vi "SMSsendCommand.vi"(0 "HULK SMS address in":refnum<visa-resource-name>, 1 "SMS controls":T1, 5 "error in":errorcluster, 6 "MID field value":dbl, 7 "Voltage limit":dbl, 8 "MAX field value":dbl, 9 "Set heater (V)":dbl, 10 "RAMP rate":dbl, 11 "Field constant (Tesla/Amp)":dbl) -> (14 "HULK SMS address out":refnum<visa-resource-name>, 17 "return count":u32, 19 "error out":errorcluster)   [LabVIEW 2017]
uses:
  SMScontrols.ctl
panel:
  out "concatenated string":string
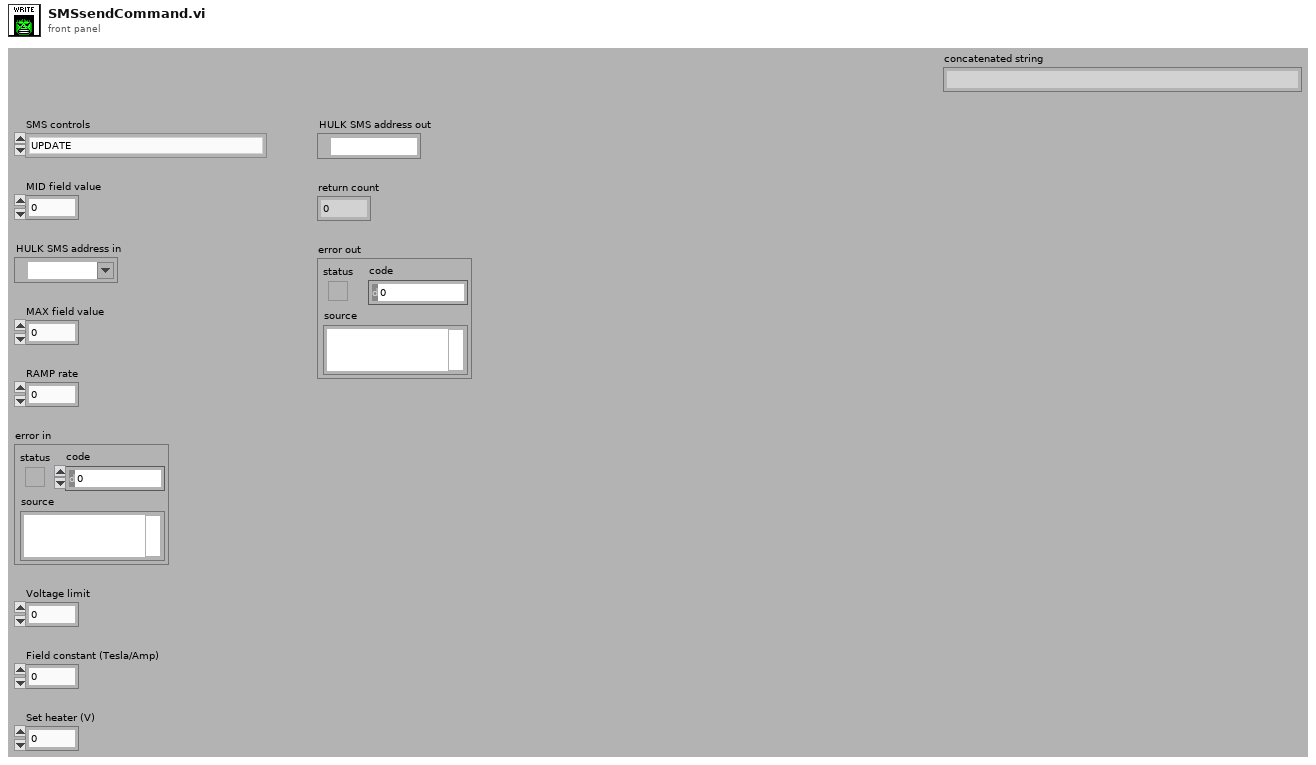
[diagram p1: front panel]
types:
  T1 = typedef "SMScontrols.ctl" = enum16{"UPDATE", "GET OUTPUT", "RAMP ZERO", "RAMP MID", "RAMP MAX", "RAMP STATUS", "PAUSE OFF", "PAUSE ON", "HEATER OFF", "HEATER ON", "TESLA OFF", "TESLA ON", "DIRECTION +", "DIRECTION -", "DIRECTION 0", "SET MID", "SET MAX", "SET RAMP", "SET LIMIT", "SET TPA", "SET HEATER"}
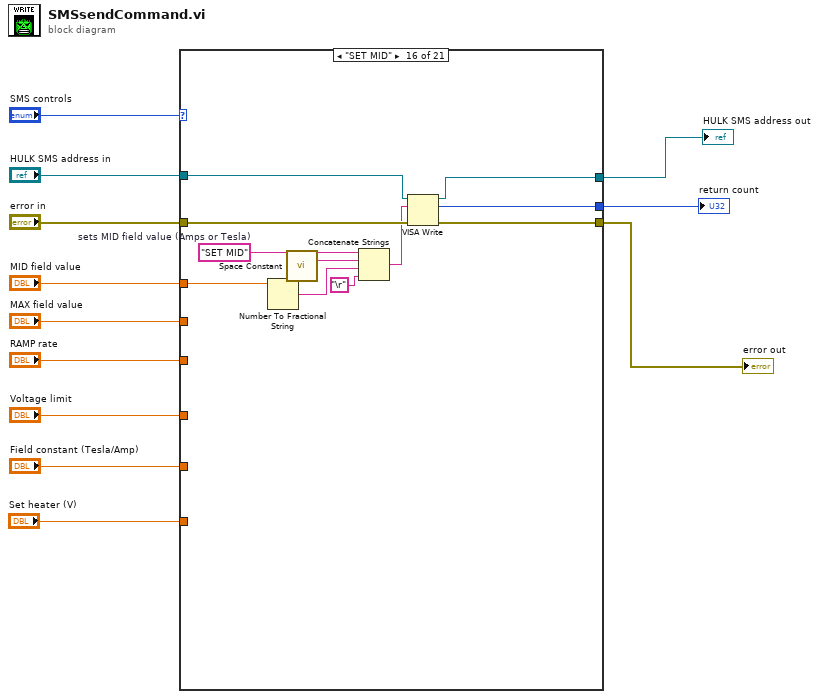
[diagram p0: block diagram]
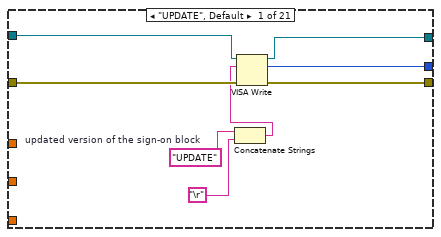
[diagram p2: hidden frame]
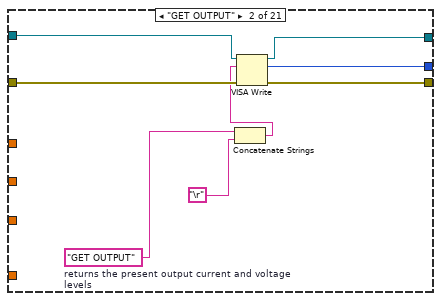
[diagram p3: hidden frame]
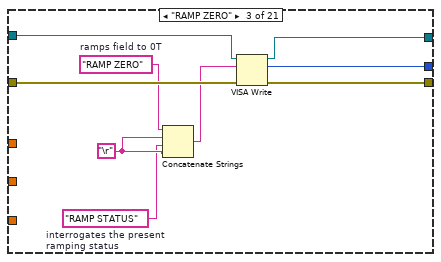
[diagram p4: hidden frame]
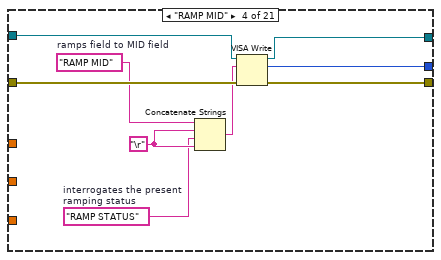
[diagram p5: hidden frame]
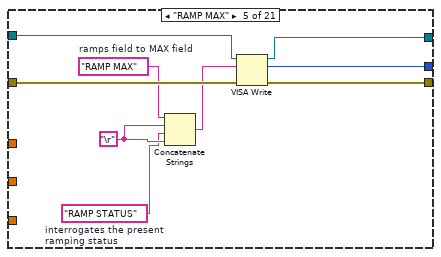
[diagram p6: hidden frame]
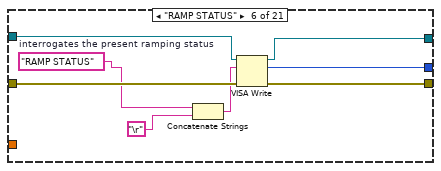
[diagram p7: hidden frame]
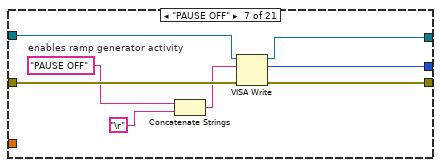
[diagram p8: hidden frame]
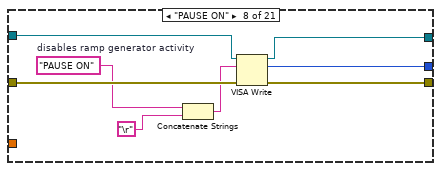
[diagram p9: hidden frame]
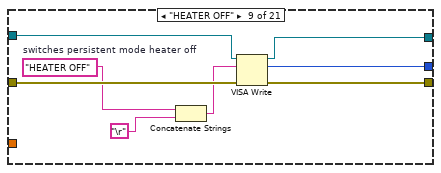
[diagram p10: hidden frame]
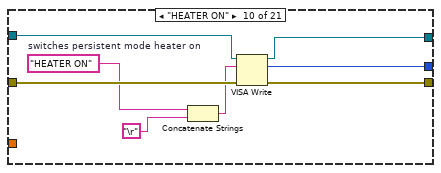
[diagram p11: hidden frame]
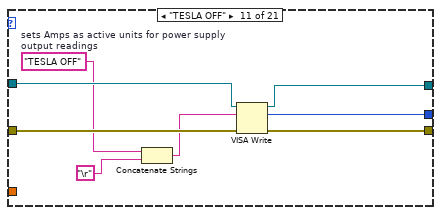
[diagram p12: hidden frame]
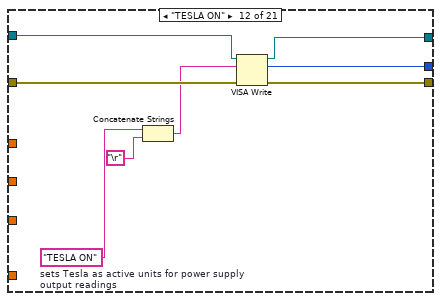
[diagram p13: hidden frame]
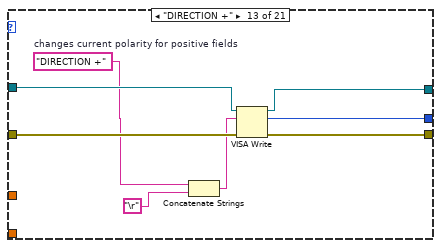
[diagram p14: hidden frame]
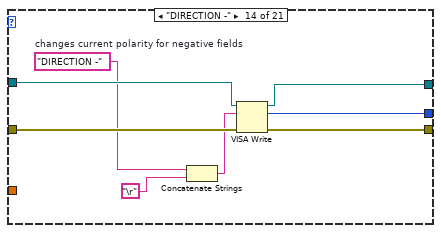
[diagram p15: hidden frame]
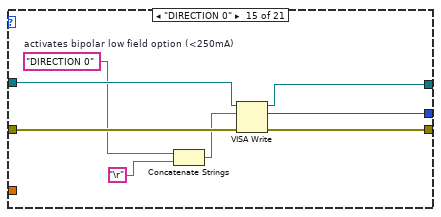
[diagram p16: hidden frame]
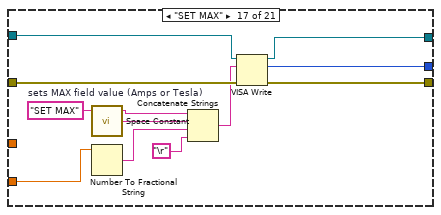
[diagram p17: hidden frame]
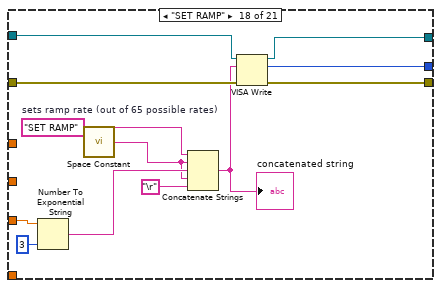
[diagram p18: hidden frame]
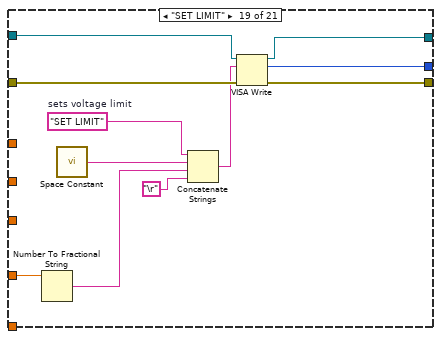
[diagram p19: hidden frame]
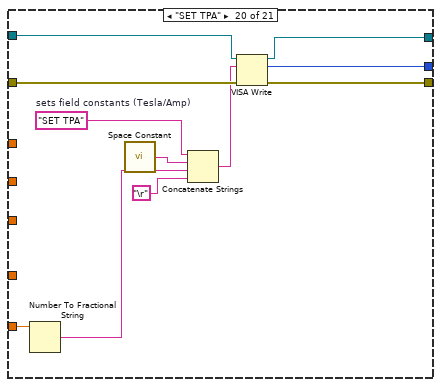
[diagram p20: hidden frame]
diagram:
  n1 = case shown="\"SET MID\"" "SMS controls" {
    tunnel: "HULK SMS address in" -> [w20 w28 w37 w46 w55 w63 w71 w79 w87 w95 w103 w111 w119 w127 w135 w146 w157 w169 w180 w191 w202]
    tunnel: [w19 w27 w36 w45 w54 w62 w70 w78 w86 w94 w102 w110 w118 w126 w134 w145 w156 w168 w179 w190 w201] -> w3
    tunnel: "error in" -> [w18 w26 w35 w44 w53 w61 w69 w77 w85 w93 w101 w109 w117 w125 w133 w144 w155 w167 w178 w189 w200]
    tunnel: [w17 w25 w34 w43 w52 w60 w68 w76 w84 w92 w100 w108 w116 w124 w132 w143 w154 w166 w177 w188 w199] -> w5
    tunnel: [w16 w24 w33 w42 w51 w59 w67 w75 w83 w91 w99 w107 w115 w123 w131 w142 w153 w165 w176 w187 w198] -> w6
    tunnel: "MID field value" -> [_ _ _ _ _ _ _ _ _ _ _ _ _ _ _ w138 _ _ _ _ _]
    tunnel: "MAX field value" -> [_ _ _ _ _ _ _ _ _ _ _ _ _ _ _ _ w148 _ _ _ _]
    tunnel: "RAMP rate" -> [_ _ _ _ _ _ _ _ _ _ _ _ _ _ _ _ _ w161 _ _ _]
    tunnel: "Voltage limit" -> [_ _ _ _ _ _ _ _ _ _ _ _ _ _ _ _ _ _ w171 _ _]
    tunnel: "Field constant (Tesla/Amp)" -> [_ _ _ _ _ _ _ _ _ _ _ _ _ _ _ _ _ _ _ w182 _]
    tunnel: "Set heater (V)" -> [_ _ _ _ _ _ _ _ _ _ _ _ _ _ _ _ _ _ _ _ w193]
    frame "UPDATE", Default {
      w15 = "UPDATE"  # updated version of the sign-on block
      n2 = Concatenate Strings(w15, "\r") -> (w13:string)
      n3 = VISA Write(VISA resource name=w20, write buffer=w13, error in (no error)=w18) -> (VISA resource name out=w17:refnum<visa-resource-name>, return count=w16:u32, error out=w19:errorcluster)
    }
    frame "GET OUTPUT" {
      w21 = "GET OUTPUT"  # returns the present output current and voltage levels
      n4 = Concatenate Strings(w21, "\r") -> (w22:string)
      n5 = VISA Write(VISA resource name=w28, write buffer=w22, error in (no error)=w26) -> (VISA resource name out=w25:refnum<visa-resource-name>, return count=w24:u32, error out=w27:errorcluster)
    }
    frame "RAMP ZERO" {
      w29 = "RAMP STATUS"  # interrogates the present ramping status
      w30 = "\r"
      w32 = "RAMP ZERO"  # ramps field to 0T
      n6 = Concatenate Strings(w32, w30, w29, w30) -> (w31:string)
      n7 = VISA Write(VISA resource name=w37, write buffer=w31, error in (no error)=w35) -> (VISA resource name out=w34:refnum<visa-resource-name>, return count=w33:u32, error out=w36:errorcluster)
    }
    frame "RAMP MID" {
      w38 = "RAMP STATUS"  # interrogates the present ramping status
      w39 = "\r"
      w41 = "RAMP MID"  # ramps field to MID field
      n8 = Concatenate Strings(w41, w39, w38, w39) -> (w40:string)
      n9 = VISA Write(VISA resource name=w46, write buffer=w40, error in (no error)=w44) -> (VISA resource name out=w43:refnum<visa-resource-name>, return count=w42:u32, error out=w45:errorcluster)
    }
    frame "RAMP MAX" {
      w47 = "RAMP STATUS"  # interrogates the present ramping status
      w48 = "\r"
      w50 = "RAMP MAX"  # ramps field to MAX field
      n10 = Concatenate Strings(w50, w48, w47, w48) -> (w49:string)
      n11 = VISA Write(VISA resource name=w55, write buffer=w49, error in (no error)=w53) -> (VISA resource name out=w52:refnum<visa-resource-name>, return count=w51:u32, error out=w54:errorcluster)
    }
    frame "RAMP STATUS" {
      w57 = "RAMP STATUS"  # interrogates the present ramping status
      n12 = Concatenate Strings(w57, "\r") -> (w56:string)
      n13 = VISA Write(VISA resource name=w63, write buffer=w56, error in (no error)=w61) -> (VISA resource name out=w60:refnum<visa-resource-name>, return count=w59:u32, error out=w62:errorcluster)
    }
    frame "PAUSE OFF" {
      w65 = "PAUSE OFF"  # enables ramp generator activity
      n14 = Concatenate Strings(w65, "\r") -> (w64:string)
      n15 = VISA Write(VISA resource name=w71, write buffer=w64, error in (no error)=w69) -> (VISA resource name out=w68:refnum<visa-resource-name>, return count=w67:u32, error out=w70:errorcluster)
    }
    frame "PAUSE ON" {
      w73 = "PAUSE ON"  # disables ramp generator activity
      n16 = Concatenate Strings(w73, "\r") -> (w72:string)
      n17 = VISA Write(VISA resource name=w79, write buffer=w72, error in (no error)=w77) -> (VISA resource name out=w76:refnum<visa-resource-name>, return count=w75:u32, error out=w78:errorcluster)
    }
    frame "HEATER OFF" {
      w81 = "HEATER OFF"  # switches persistent mode heater off
      n18 = Concatenate Strings(w81, "\r") -> (w80:string)
      n19 = VISA Write(VISA resource name=w87, write buffer=w80, error in (no error)=w85) -> (VISA resource name out=w84:refnum<visa-resource-name>, return count=w83:u32, error out=w86:errorcluster)
    }
    frame "HEATER ON" {
      w89 = "HEATER ON"  # switches persistent mode heater on
      n20 = Concatenate Strings(w89, "\r") -> (w88:string)
      n21 = VISA Write(VISA resource name=w95, write buffer=w88, error in (no error)=w93) -> (VISA resource name out=w92:refnum<visa-resource-name>, return count=w91:u32, error out=w94:errorcluster)
    }
    frame "TESLA OFF" {
      w97 = "TESLA OFF"  # sets Amps as active units for power supply output readings
      n22 = Concatenate Strings(w97, "\r") -> (w96:string)
      n23 = VISA Write(VISA resource name=w103, write buffer=w96, error in (no error)=w101) -> (VISA resource name out=w100:refnum<visa-resource-name>, return count=w99:u32, error out=w102:errorcluster)
    }
    frame "TESLA ON" {
      w105 = "TESLA ON"  # sets Tesla as active units for power supply output readings
      n24 = Concatenate Strings(w105, "\r") -> (w104:string)
      n25 = VISA Write(VISA resource name=w111, write buffer=w104, error in (no error)=w109) -> (VISA resource name out=w108:refnum<visa-resource-name>, return count=w107:u32, error out=w110:errorcluster)
    }
    frame "DIRECTION +" {
      w113 = "DIRECTION +"  # changes current polarity for positive fields
      n26 = Concatenate Strings(w113, "\r") -> (w112:string)
      n27 = VISA Write(VISA resource name=w119, write buffer=w112, error in (no error)=w117) -> (VISA resource name out=w116:refnum<visa-resource-name>, return count=w115:u32, error out=w118:errorcluster)
    }
    frame "DIRECTION -" {
      w121 = "DIRECTION -"  # changes current polarity for negative fields
      n28 = Concatenate Strings(w121, "\r") -> (w120:string)
      n29 = VISA Write(VISA resource name=w127, write buffer=w120, error in (no error)=w125) -> (VISA resource name out=w124:refnum<visa-resource-name>, return count=w123:u32, error out=w126:errorcluster)
    }
    frame "DIRECTION 0" {
      w129 = "DIRECTION 0"  # activates bipolar low field option (<250mA)
      n30 = Concatenate Strings(w129, "\r") -> (w128:string)
      n31 = VISA Write(VISA resource name=w135, write buffer=w128, error in (no error)=w133) -> (VISA resource name out=w132:refnum<visa-resource-name>, return count=w131:u32, error out=w134:errorcluster)
    }
    frame "SET MID" {
      w141 = "SET MID"  # sets MID field value (Amps or Tesla)
      n32 = Number To Fractional String(number=w138) -> (F-format string=w137:string)  [unwired: 3 in]
      n33 = call <vilib>:"Space Constant.vi"() -> ("String"=w140:string)
      n34 = Concatenate Strings(w141, w140, w137, "\r") -> (w139:string)
      n35 = VISA Write(VISA resource name=w146, write buffer=w139, error in (no error)=w144) -> (VISA resource name out=w143:refnum<visa-resource-name>, return count=w142:u32, error out=w145:errorcluster)
    }
    frame "SET MAX" {
      w149 = "SET MAX"  # sets MAX field value (Amps or Tesla)
      n36 = call <vilib>:"Space Constant.vi"() -> ("String"=w152:string)
      n37 = Number To Fractional String(number=w148) -> (F-format string=w150:string)  [unwired: 3 in]
      n38 = Concatenate Strings(w149, w152, w150, "\r") -> (w151:string)
      n39 = VISA Write(VISA resource name=w157, write buffer=w151, error in (no error)=w155) -> (VISA resource name out=w154:refnum<visa-resource-name>, return count=w153:u32, error out=w156:errorcluster)
    }
    frame "SET RAMP" {
      w162 = "SET RAMP"  # sets ramp rate (out of 65 possible rates)
      n40 = Number To Exponential String(number=w161, precision (6)=i16 3) -> (E-format string=w163:string)  [unwired: 2 in]
      n41 = call <vilib>:"Space Constant.vi"() -> ("String"=w159:string)
      n42 = Concatenate Strings(w162, w159, w163, w159, "\r") -> (w164:string)
      "concatenated string" <- w164
      n43 = VISA Write(VISA resource name=w169, write buffer=w164, error in (no error)=w167) -> (VISA resource name out=w166:refnum<visa-resource-name>, return count=w165:u32, error out=w168:errorcluster)
    }
    frame "SET LIMIT" {
      w172 = "SET LIMIT"  # sets voltage limit
      n44 = Number To Fractional String(number=w171) -> (F-format string=w173:string)  [unwired: 3 in]
      n45 = call <vilib>:"Space Constant.vi"() -> ("String"=w175:string)
      n46 = Concatenate Strings(w172, w175, w173, "\r") -> (w174:string)
      n47 = VISA Write(VISA resource name=w180, write buffer=w174, error in (no error)=w178) -> (VISA resource name out=w177:refnum<visa-resource-name>, return count=w176:u32, error out=w179:errorcluster)
    }
    frame "SET TPA" {
      w183 = "SET TPA"  # sets field constants (Tesla/Amp)
      n48 = Number To Fractional String(number=w182) -> (F-format string=w184:string)  [unwired: 3 in]
      n49 = call <vilib>:"Space Constant.vi"() -> ("String"=w186:string)
      n50 = Concatenate Strings(w183, w186, w184, "\r") -> (w185:string)
      n51 = VISA Write(VISA resource name=w191, write buffer=w185, error in (no error)=w189) -> (VISA resource name out=w188:refnum<visa-resource-name>, return count=w187:u32, error out=w190:errorcluster)
    }
    frame "SET HEATER" {
      w194 = "SET HEATER"  # sets heater output (Volts)
      n52 = Number To Fractional String(number=w193) -> (F-format string=w195:string)  [unwired: 3 in]
      n53 = call <vilib>:"Space Constant.vi"() -> ("String"=w197:string)
      n54 = Concatenate Strings(w194, w197, w195, "\r") -> (w196:string)
      n55 = VISA Write(VISA resource name=w202, write buffer=w196, error in (no error)=w200) -> (VISA resource name out=w199:refnum<visa-resource-name>, return count=w198:u32, error out=w201:errorcluster)
    }
  }
  "return count" <- w6
  "HULK SMS address out" <- w5
  "error out" <- w3
